vi "Backup.vi"(8 "error in (no error)":errorcluster, 11 "JSON Lexer in":refnum<class "JSON Lexer.lvclass">) -> (0 "error out":errorcluster, 3 "JSON Lexer out":refnum<class "JSON Lexer.lvclass">)   [LabVIEW 2013, in "JKI JSON Serialization.lvlib" / "JSON Lexer.lvclass"]
uses:
  JSON Lexer.lvclass
  JSON Lexer.lvclass/JSON Lexer.ctl
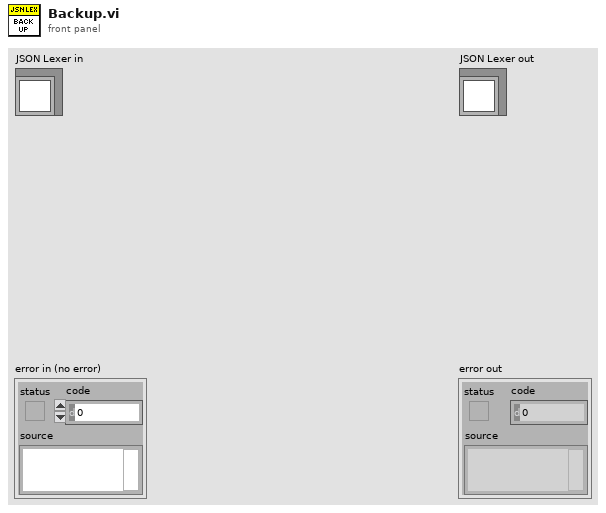
[diagram p1: front panel]
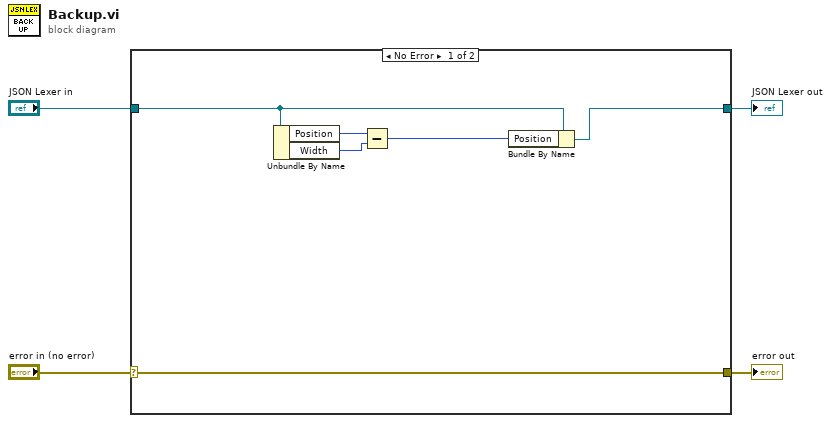
[diagram p0: block diagram]
diagram:
  n1 = case shown="No Error" "error in (no error)" {
    selector: "error in (no error)" -> [w5 w12]
    tunnel: [w5 w12] -> w3
    tunnel: [w9 w11] -> w1
    tunnel: "JSON Lexer in" -> [w10 w11]
    frame No Error {
      n2 = Unbundle By Name(w10) -> ("Position"=w8:i32, "Width"=w7:i32)
      n3 = Subtract(x=w8, y=w7) -> (x-y=w6:i32)
      n4 = Bundle By Name(cluster=w10, "Position"=w6) -> (w9:refnum<class "JSON Lexer.lvclass">)
    }
    frame Error {
    }
  }
  "error out" <- w3
  "JSON Lexer out" <- w1
